vi "cbc radio label parse.vi"(8 "error in (no error)":errorcluster) -> (0 "error out":errorcluster, 1 "Radio Model":string, 2 "All good generic?":bool, 3 "All good Duke?":bool, 4 "Eight CSV items":string[](array[string]))   [LabVIEW 2013]
panel:
  in  "Exit":bool
  out "Is Duke label?":bool
  out "IP addr good?":bool
  out "Phone OK?":bool
  out "Valid model?":bool
  out "Valid SN?":bool
  out "Valid SimId?":bool
  out "Valid IMEI?":bool
  out "Have all 8 fields?":bool
  in  "String to parse with commas":string
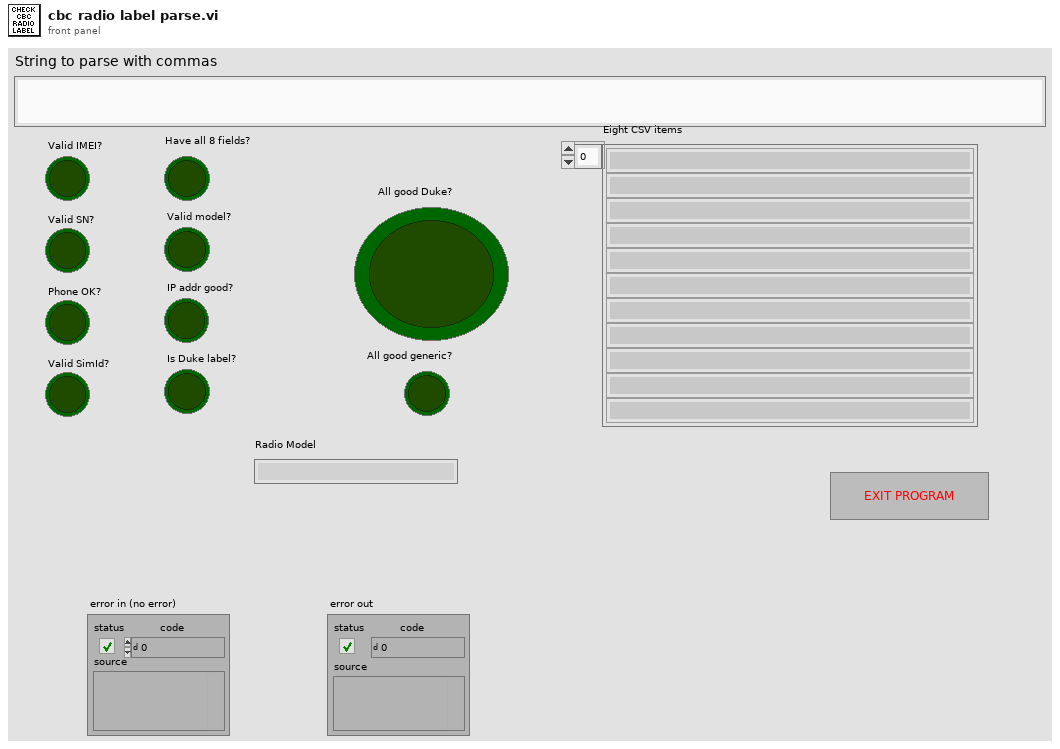
[diagram p1: front panel]
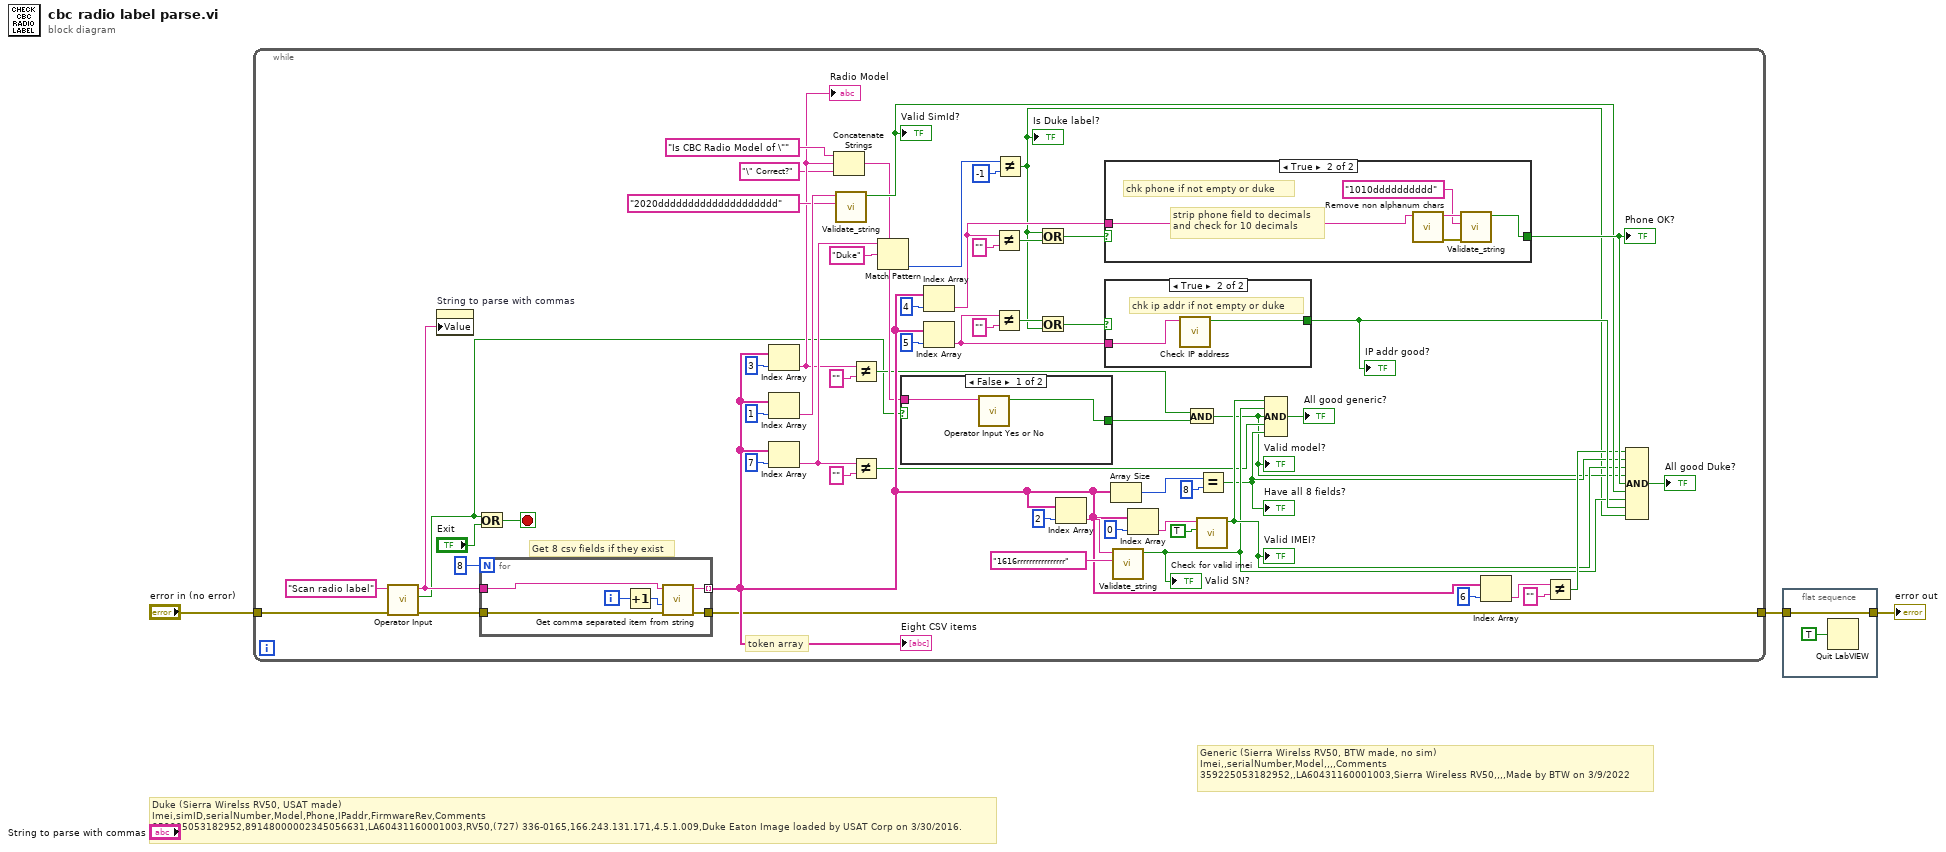
[diagram p0: block diagram]
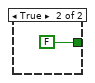
[diagram p2: hidden frame]
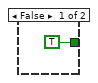
[diagram p3: hidden frame]
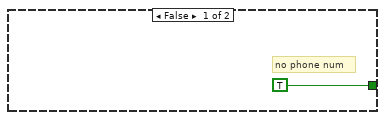
[diagram p4: hidden frame]
diagram:
  # "Generic (Sierra Wirelss RV50, BTW made, no sim)\nImei,,serialNumber,Model,,,,Comments\n359225053182952,,LA60431160001003,Sierra Wireless RV50,,,,Made by BTW on 3/9/2022"
  # "Duke (Sierra Wirelss RV50, USAT made)\nImei,simID,serialNumber,Model,Phone,IPaddr,FirmwareRev,Comments\n359225053182952,89148000002345056631,LA60431160001003,RV50,(727) 336-0165,166.243.131.171,4.5.1.009,Duke Eaton Image loaded by USAT Corp on 3/30/2016."
  n1 = while {
    tunnel: "error in (no error)" -> [w61]
    tunnel: [w12] -> w1
    stop <- w10 stop-if-true
    # "token array"
    # "Get 8 csv fields if they exist"
    n2 = call "Operator Input.vi"("error in (no error)"=w61, "Message"="Scan radio label") -> ("error out"=w60:errorcluster, "Stop button hit"=w9:bool, "Response"=w36:string)  [unwired: 7 in]
    n3 = property on="String to parse with commas" class="Str"("Value"=w36) -> ()  [unwired: 2 in, 2 out]
    n4 = Or(x=w9, y="Exit") -> (x .or. y?=w10:bool)
    n5 = for {
      N: 8 -> [_]
      tunnel: w60 -> [w81]
      tunnel: [w80] -> w12
      tunnel: [w77] -> w29 mode=indexing
      tunnel: w36 -> [w76]
      i -> [w79]
      n6 = Increment(x=w79) -> (x+1=w78:i32)
      n7 = call "Get comma separated item from string.vi"("error in (no error)"=w81, "Field Num (1-n)"=w78, "String to parse with commas"=w76) -> ("error out"=w80:errorcluster, "Item string value"=w77:string)  [unwired: 7 in]
    }
    "Eight CSV items" <- w29
    n8 = Index Array(array=w29, index=3) -> (element=w18:string)
    "Radio Model" <- w18
    n9 = Index Array(array=w29, index=1) -> (element=w53:string)
    n10 = Index Array(array=w29, index=7) -> (element=w24:string)
    n11 = Concatenate Strings("Is CBC Radio Model of \"" ("Operator text"), w18, "\" Correct?" ("string")) -> (w16:string)
    n12 = call "Validate_string.vi"("String data format"="2020dddddddddddddddddddd", "String"=w53) -> ("String Valid"=w40:bool)  [unwired: 8 in, 1 out]
    "Valid SimId?" <- w40
    n13 = Not Equal?(x=w18, y="") -> (x != y?=w15:bool)
    n14 = Not Equal?(x=w24, y="") -> (x != y?=w22:bool)
    n15 = Match Pattern(string=w24, regular expression="Duke") -> (offset past match=w33:i32)  [unwired: 1 in, 3 out]
    n16 = case shown="False" w9 {
      tunnel: w16 -> [w65 _]
      tunnel: [w64 FALSE ("Yes clicked")] -> w13
      frame False {
        n17 = call "Operator Input Yes or No.vi"("Operator text"=w65) -> ("Yes clicked"=w64:bool)  [unwired: 8 in, 2 out]
      }
      frame True {
      }
    }
    n18 = Index Array(array=w29, index=4) -> (element=w44:string)
    n19 = Index Array(array=w29, index=5) -> (element=w39:string)
    n20 = Not Equal?(x=w44, y="") -> (x != y?=w6:bool)
    n21 = Not Equal?(x=w39, y="") -> (x != y?=w8:bool)
    n22 = Not Equal?(x=w33, y=-1) -> (x != y?=w4:bool)
    "Is Duke label?" <- w4
    n23 = Or(x=w4, y=w6) -> (x .or. y?=w5:bool)
    n24 = Or(x=w8, y=w4) -> (x .or. y?=w7:bool)
    n25 = Index Array(array=w29, index=2) -> (element=w50:string)
    n26 = case shown="True" w5 {
      tunnel: w44 -> [_ w75]
      tunnel: [TRUE ("String Valid") w71] -> w41
      frame False {
        # "no phone num"
      }
      frame True {
        # "chk phone if not empty or duke"
        # "strip phone field to decimals\nand check for 10 decimals"
        n27 = call "Remove non alphanum chars.vi"("String In"=w75) -> ("error out"=w74:errorcluster, "String Out"=w73:string)  [unwired: 9 in]
        n28 = call "Validate_string.vi"("error in (no error)"=w74, "String data format"="1010dddddddddd", "String"=w73) -> ("String Valid"=w71:bool)  [unwired: 7 in, 1 out]
      }
    }
    "Phone OK?" <- w41
    n29 = case shown="True" w7 {
      tunnel: w39 -> [_ w69]
      tunnel: [TRUE ("Got all fields and data good?") w68] -> w38
      frame False {
      }
      frame True {
        # "chk ip addr if not empty or duke"
        n30 = call "Check IP address.vi"("IP string"=w69) -> ("Got all fields and data good?"=w68:bool)  [unwired: 9 in, 1 out]
      }
    }
    "IP addr good?" <- w38
    n31 = Array Size(array=w29) -> (size(s)=w59:i32)
    n32 = call "Validate_string.vi"("String data format"="1616rrrrrrrrrrrrrrrr", "String"=w50) -> ("String Valid"=w25:bool)  [unwired: 8 in, 1 out]
    "Valid SN?" <- w25
    n33 = Index Array(array=w29, index=0) -> (element=w56:string)
    n34 = And(x=w15, y=w13) -> (x .and. y?=w14:bool)
    "Valid model?" <- w14
    n35 = call "Check for valid imei.vi"("Got Imei?"=TRUE, "14 or 15 digit IMEI"=w56) -> ("Valid IMEI"=w26:bool)  [unwired: 7 in, 2 out]
    "Valid IMEI?" <- w26
    n36 = Equal?(x=w59, y=8) -> (x = y?=w20:bool)
    "Have all 8 fields?" <- w20
    n37 = Compound Arithmetic op=AND(w26, w25, w14, w22, w20) -> (→"All good generic?":bool)
    n38 = Index Array(array=w29, index=6) -> (element=w28:string)
    n39 = Not Equal?(x=w28, y="") -> (x != y?=w27:bool)
    n40 = Compound Arithmetic op=AND(w27, w20, w26, w14, w41, w40, w25, w38, w4) -> (→"All good Duke?":bool)
  }
  n41 = flat-sequence {
    tunnel: [w83] -> w2
    tunnel: w1 -> [w83]
    frame #0 {
      n42 = Quit LabVIEW(quit? (T)=TRUE) -> ()
    }
  }
  "error out" <- w2
